vi "updateTimer.vi"(8 "error in (no error)":errorcluster, 11 "Heartbeat in":refnum<class "Heartbeat.lvclass">) -> (0 "error out":errorcluster, 2 "getStatus?":bool, 3 "Heartbeat out":refnum<class "Heartbeat.lvclass">)   [LabVIEW 2016, in "Heartbeat.lvclass"]
uses:
  Heartbeat.lvclass
  Heartbeat.lvclass/Heartbeat.ctl
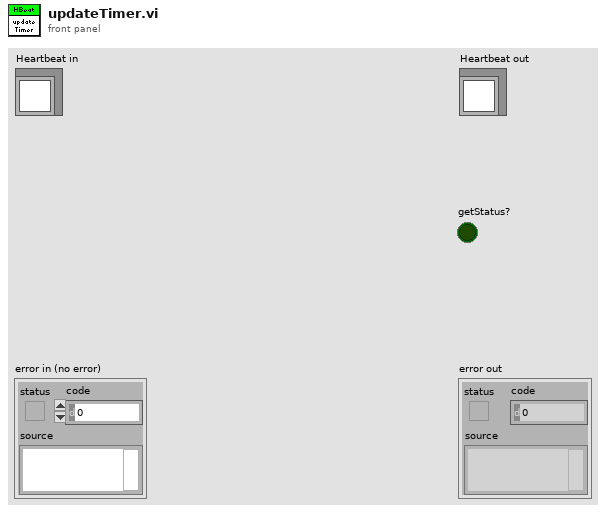
[diagram p1: front panel]
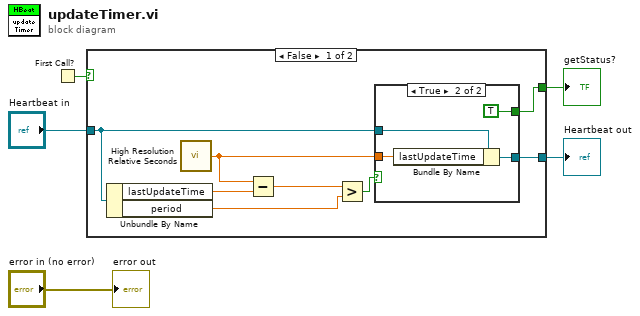
[diagram p0: block diagram]
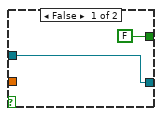
[diagram p2: hidden frame]
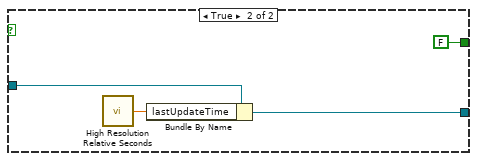
[diagram p3: hidden frame]
diagram:
  n1 = First Call?() -> (First Call?: T/F=w4:bool)
  n2 = case shown="False" w4 {
    tunnel: "Heartbeat in" -> [w9 w23]
    tunnel: [w8 w22] -> w2
    tunnel: [w7 FALSE ("getStatus?")] -> w5
    frame False {
      n3 = Unbundle By Name(w9) -> ("lastUpdateTime"=w13:dbl, "period"=w11:dbl)
      n4 = call <vilib>:"High Resolution Relative Seconds.vi"() -> ("relative seconds"=w6:dbl)
      n5 = Subtract(x=w6, y=w13) -> (x-y=w12:dbl)
      n6 = Greater?(x=w12, y=w11) -> (0:w10:bool)
      n7 = case shown="True" w10 {
        tunnel: w9 -> [w15 w18]
        tunnel: [w15 w16] -> w8
        tunnel: [FALSE ("getStatus?") TRUE ("getStatus?")] -> w7
        tunnel: w6 -> [_ w17]
        frame False {
        }
        frame True {
          n8 = Bundle By Name(cluster=w18, "lastUpdateTime"=w17) -> (w16:refnum<class "Heartbeat.lvclass">)
        }
      }
    }
    frame True {
      n9 = call <vilib>:"High Resolution Relative Seconds.vi"() -> ("relative seconds"=w20:dbl)
      n10 = Bundle By Name(cluster=w23, "lastUpdateTime"=w20) -> (w22:refnum<class "Heartbeat.lvclass">)
    }
  }
  "Heartbeat out" <- w2
  "getStatus?" <- w5
  "error out" <- "error in (no error)"
